vi "Cleanup Module.vi"(8 "error in (no error)":errorcluster, 11 "Event Reporter Module in":refnum<class "Event Reporter Module.lvclass">) -> (0 "error out":errorcluster, 3 "Event Reporter Module out":refnum<class "Event Reporter Module.lvclass">)   [LabVIEW 2020, in "Volatus.lvlib" / "Event Reporter Module.lvclass"]
uses:
  Event Reporter Module.lvclass
  Event Reporter Module.lvclass/Event Reporter Module.ctl
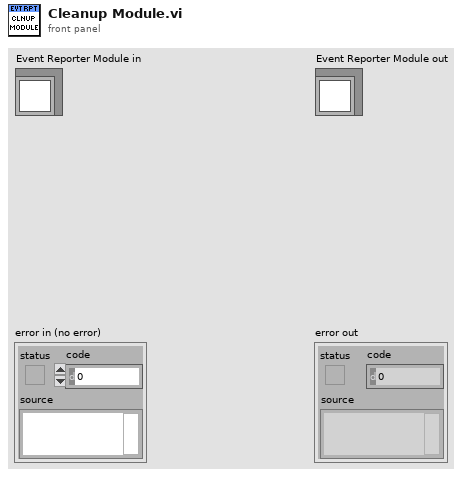
[diagram p1: front panel]
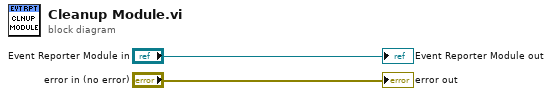
[diagram p0: block diagram]
diagram:
  "error out" <- "error in (no error)"
  "Event Reporter Module out" <- "Event Reporter Module in"
